vi "_PC_Pub_Splitter_ToolbarWindow.vi"(1 "sys_value_list":refnum<vi>, 2 "d999_list":refnum<vi>, 3 "Config Tab":refnum<vi>, 4 "SplitterRef":refnum<vi>) -> ()   [LabVIEW 2018]
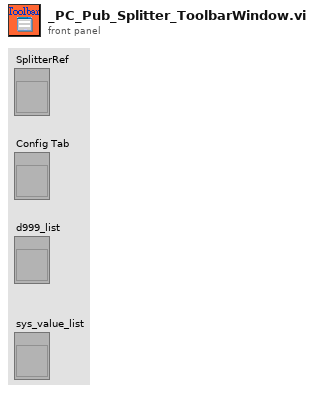
[diagram p1: front panel]
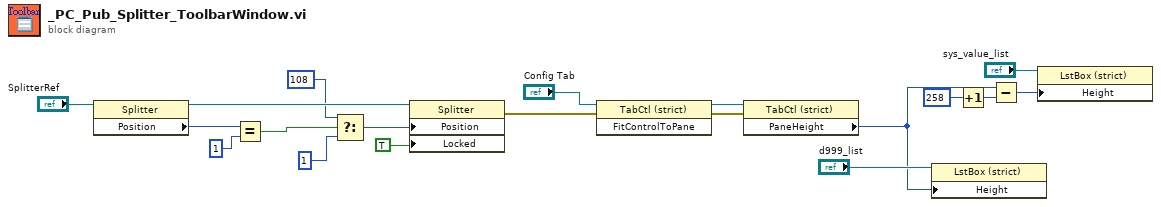
[diagram p0: block diagram]
diagram:
  n1 = property class="Splitter"(reference="SplitterRef") -> (reference out=w19:refnum<vi>, "Position"=w14:i32)  [unwired: 1 in, 1 out]
  n2 = Equal?(x=w14, y=1) -> (x = y?=w11:bool)
  n3 = Select(t=108 ("Splitter Position"), s=w11, f=1) -> (s? t:f=w13:i32)
  n4 = property class="Splitter"(reference=w19, "Position"=w13, "Locked"=TRUE ("Splitter Position Locked")) -> (error out=w10:errorcluster)  [unwired: 1 in, 1 out]
  n5 = invoke class="TabCtl (strict)" method="FitControlToPane"(reference="Config Tab", error in=w10) -> (reference out=w8:refnum<vi>, error out=w9:errorcluster)  [unwired: 1 in, 1 out]
  n6 = property class="TabCtl (strict)"(reference=w8, error in=w9) -> ("PaneHeight"=w3:u32)  [unwired: 2 out]
  n7 = property class="LstBox (strict)"(reference="d999_list", "Height"=w3) -> ()  [unwired: 1 in, 2 out]
  n8 = Increment(x=u32 258 ("Height")) -> (x+1=w1:u32)
  n9 = Subtract(x=w3, y=w1) -> (x-y=w2:u32)
  n10 = property class="LstBox (strict)"(reference="sys_value_list", "Height"=w2) -> ()  [unwired: 1 in, 2 out]
